vi "Exit.vi"   [LabVIEW 2015]
uses:
  ESLSCDLL.dll
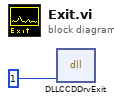
[diagram p0: block diagram]
diagram:
  n1 = dll-call lib="C:/Users/Gerhard/Desktop/testlv15/board.vis/ESLSCDLL.dll" fn="DLLCCDDrvExit"("drv"=u32 1) -> ()  [unwired: 5 in, 2 out]
